vi "get_all_string_constants_of_VI.vi"(11 "VI_path":path) -> (2 "VI_name":string, 3 "string_constants":string[](array[string]))   [LabVIEW 2019]
uses:
  <vilib>/Utility/traverseref.llb/TRef TravTarget.ctl
  <vilib>/Utility/traverseref.llb/VI Scripting - Traverse.lvlib
  <vilib>/Utility/Data Type/NI_Data Type.lvlib
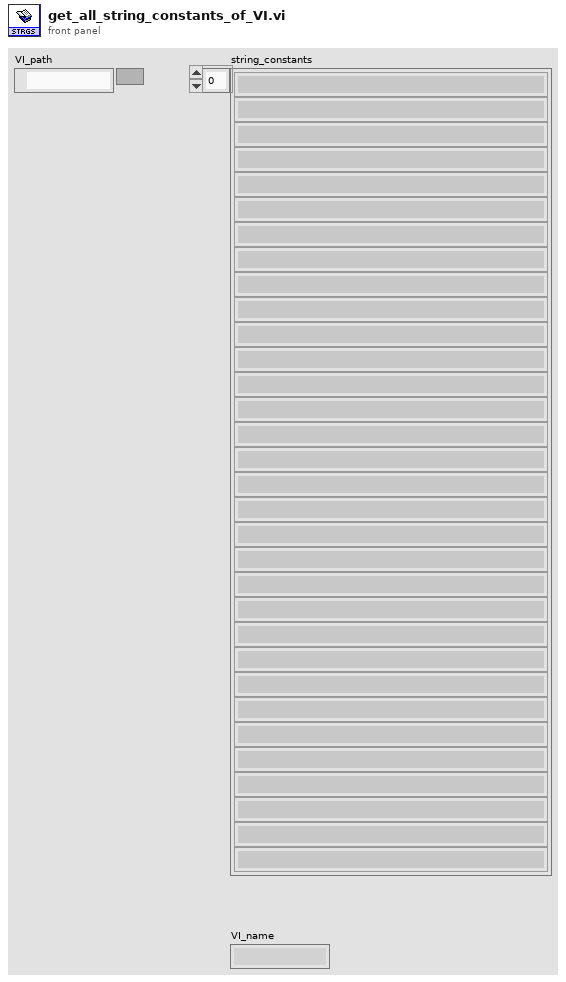
[diagram p1: front panel]
types:
  T1 = typedef "TRef TravTarget.ctl" = enum16{"FP", "BD", "Other"}
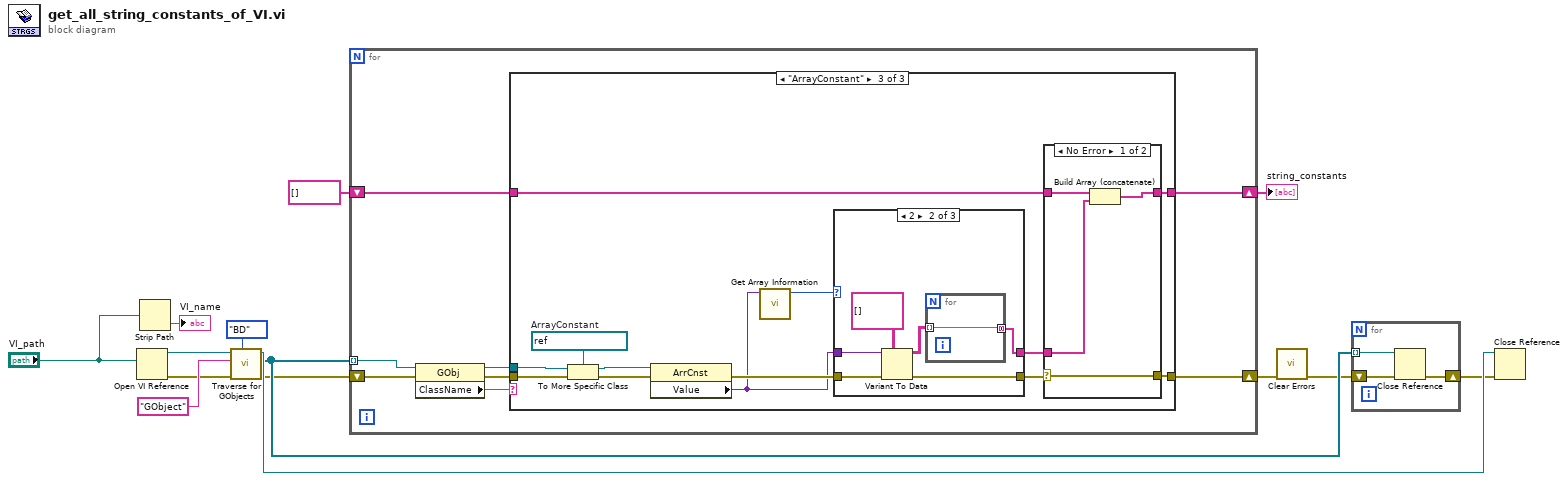
[diagram p0: block diagram]
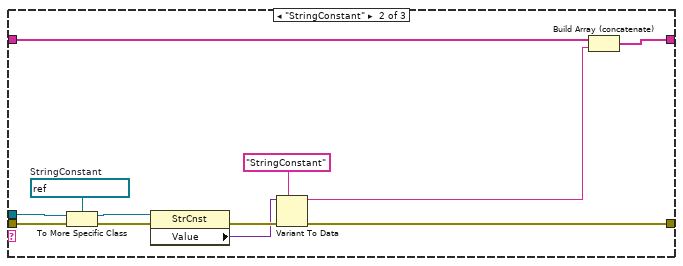
[diagram p3: hidden frame]
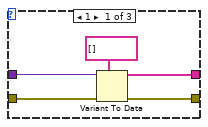
[diagram p4: hidden frame]
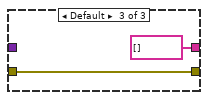
[diagram p5: hidden frame]
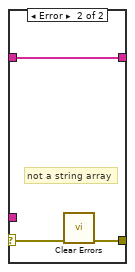
[diagram p6: hidden frame]
diagram:
  n1 = Open VI Reference(vi path="VI_path") -> (vi reference=w12:refnum<vi>, error out=w3:errorcluster)  [unwired: 5 in]
  n2 = Strip Path(path="VI_path") -> (name=→"VI_name":string)  [unwired: 1 out]
  n3 = call <vilib>:"Traverse for GObjects.vi"("Traverse Target"=TRef_TravTarget."BD", "error in (no error)"=w3, "Class Name"="GObject", "VI Refnum"=w12) -> ("error out"=w5:errorcluster, "References"=w6:refnum<vi>[], "dup VI Refnum"=w8:refnum<vi>)  [unwired: 4 in, 1 out]
  n4 = for {
    tunnel: w6 -> [w22] mode=indexing
    shift-right: [w18] -> w2
    shift-left: w5 -> [w21]
    shift-right: [w16] -> w9
    shift-left: string[] [] -> [w15]
    n5 = property class="GObj"(reference=w22, error in=w21) -> (reference out=w17:refnum<vi>, error out=w19:errorcluster, "ClassName"=w20:string)
    n6 = case shown="\"ArrayConstant\"" w20 {
      tunnel: w19 -> [w23 w33 w46]
      tunnel: [w23 w30 w42] -> w18
      tunnel: w17 -> [_ w36 w49]
      tunnel: [w24 w27 w44] -> w16
      tunnel: w15 -> [w24 w26 w43]
      frame Default {
      }
      frame "StringConstant" {
        w34 = refnum<vi> refnum  # StringConstant
        n7 = To More Specific Class(target class=w34, reference=w36, error in=w33) -> (specific class reference=w35:refnum<vi>, error out=w32:errorcluster)
        n8 = property class="StrCnst"(reference=w35, error in=w32) -> (error out=w31:errorcluster, "Value"=w29:variant)  [unwired: 1 out]
        n9 = Variant To Data(error in=w31, type="StringConstant", Variant=w29) -> (data=w28:string, error out=w30:errorcluster)
        n10 = Build Array (concatenate)(w26, w28) -> (w27:string[])
      }
      frame "ArrayConstant" {
        w47 = refnum<vi> refnum  # ArrayConstant
        n11 = To More Specific Class(target class=w47, reference=w49, error in=w46) -> (specific class reference=w48:refnum<vi>, error out=w45:errorcluster)
        n12 = property class="ArrCnst"(reference=w48, error in=w45) -> (error out=w40:errorcluster, "Value"=w39:variant)  [unwired: 1 out]
        n13 = call <vilib>:"Get Array Information.vi"("variant"=w39) -> ("number of dimensions"=w38:i32)  [unwired: 7 in, 3 out]
        n14 = case shown="2" w38 {
          tunnel: [w51 w57 w63] -> w41
          tunnel: w40 -> [w54 w60 w63]
          tunnel: w39 -> [w53 w59 _]
          tunnel: [w50 w55 string[] []] -> w37
          frame 1 {
            n15 = Variant To Data(error in=w54, type=string[] [], Variant=w53) -> (data=w50:string[], error out=w51:errorcluster)
          }
          frame 2 {
            n16 = Variant To Data(error in=w60, type=string[][] [], Variant=w59) -> (data=w56:string[][], error out=w57:errorcluster)
            n17 = for {
              tunnel: w56 -> [w61] mode=indexing
              tunnel: [w61] -> w55 mode=concatenating
            }
          }
          frame Default {
          }
        }
        n18 = case shown="No Error" w41 {
          selector: w41 -> [w64 w69]
          tunnel: w37 -> [w67 _]
          tunnel: [w66 w70] -> w44
          tunnel: w43 -> [w65 w70]
          tunnel: [w64 w68] -> w42
          frame No Error {
            n19 = Build Array (concatenate)(w65, w67) -> (w66:string[])
          }
          frame Error {
            # "not a string array"
            n20 = call <vilib>:"Clear Errors.vi"("error in (no error)"=w69) -> ("error out"=w68:errorcluster)  [unwired: 5 in, 1 out]
          }
        }
      }
    }
  }
  "string_constants" <- w9
  n21 = call <vilib>:"Clear Errors.vi"("error in (no error)"=w2) -> ("error out"=w1:errorcluster)  [unwired: 5 in, 1 out]
  n22 = for {
    shift-right: [w72] -> w7
    shift-left: w1 -> [w73]
    tunnel: w6 -> [w71] mode=indexing
    n23 = Close Reference(reference=w71, error in (no error)=w73) -> (error out=w72:errorcluster)
  }
  n24 = Close Reference(reference=w8, error in (no error)=w7) -> ()  [unwired: 1 out]
